vi "Initialize Attributes.vi"(8 "error in (no error)":errorcluster, 10 "Attribute Data":variant, 11 "PVConnection in":refnum<class "SVConnection.lvclass">) -> (0 "error out":errorcluster, 2 "Found?":bool, 3 "PVConnection out":refnum<class "SVConnection.lvclass">)   [LabVIEW 2012, in "CS++ProcessVariables.lvlib" / "SVConnection.lvclass"]
doc: "Initialize object attribute.\n\nUnique resources should be allocated elsewhere!"
uses:
  SVConnection.lvclass
  PVConnection/PVConnection.lvclass
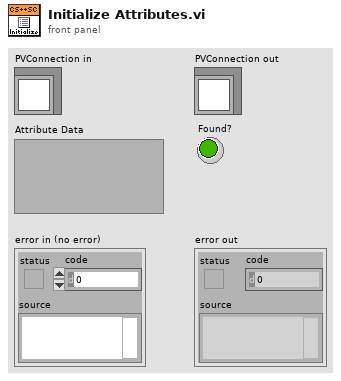
[diagram p1: front panel]
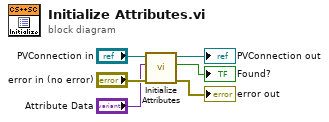
[diagram p0: block diagram]
diagram:
  n1 = call-parent "Initialize Attributes.vi"("error in (no error)"="error in (no error)", "Attribute Data"="Attribute Data", "PVConnection in"="PVConnection in") -> ("error out"=→"error out":errorcluster, "Found?"=→"Found?":bool, "PVConnection out"=→"PVConnection out":refnum<class "SVConnection.lvclass">)  [unwired: 6 in]
